vi "WLAN - TV - RW - ReadTestVectorFile(Tx).vi"(0 "TX_TV_Sequence":path[](array[path]), 5 "Measurment Settings":path[](array[path]), 13 "Index":i32) -> (4 "TV's":T2[](array[typedef]) {"Tx_Chan" format="%.0x"; "Standard" items=["80211A/G/J/P OFDM", "80211B/G DSSS", "80211G DSSSOFDM", "80211N MIMOOFDM", "80211AC MIMOOFDM"]; "OFDM Data Rate (Mbps)" items=["6", "9", "12", "18", "24", "36", "48", "54"]; "80211n PLCP Frame Format" items=["Mixed Format", "Greenfield Format"]; "FEC Coding Type" items=["BCC", "LDPC"]; "DSSS Data Rate (Mbps)" items=["1", "2", "5.5 CCK", "5.5 PBCC", "11 CCK", "11 PBCC", "22", "33"]}, 6 "Tv First Element":T2 {"Tx_Chan" format="%.0x"; "Standard" items=["80211A/G/J/P OFDM", "80211B/G DSSS", "80211G DSSSOFDM", "80211N MIMOOFDM", "80211AC MIMOOFDM"]; "OFDM Data Rate (Mbps)" items=["6", "9", "12", "18", "24", "36", "48", "54"]; "80211n PLCP Frame Format" items=["Mixed Format", "Greenfield Format"]; "FEC Coding Type" items=["BCC", "LDPC"]; "DSSS Data Rate (Mbps)" items=["1", "2", "5.5 CCK", "5.5 PBCC", "11 CCK", "11 PBCC", "22", "33"]}, 8 "Test Completed ?":bool, 10 "WLAN Measurement Settings":T3={"OFDM Advanced Controls(11ag)"={"OFDM Auto Compute Acquisition Length Enabled"=0, "OFDM Maximum Symbols Used"=0, "OFDM Time Tracking Enabled"=0, "OFDM Channel Tracking Enabled"=0, "OFDM Amplitude Tracking Enabled"=1, "OFDM CFO Estimation Method"=0, "OFDM Phase Tracking Method"=0, "OFDM Header Detection Enabled"=0, "OFDM MAC FCS Check Enabled"=0, "#Avg"=10, "#Iterations"=10}, "DSSS Demod Parameters"={"DSSS Auto Compute Acquisition Length Enabled"=0, "DSSS Equalization Enabled"=0, "DSSS Header Detection Enabled"=0, "DSSS MAC FCS Check Enabled"=0, "DSSS Measurement Start Location"=0, "DSSS Phase Tracking Method"=0, "DSSS Maximum Chips Used"=0, "DSSS Reference Pulse Shaping Filter"=0, "DSSS Reference Pulse Shaping Filter Coefficient"=0.0, "# Avg"=1024, "# Iterations"=1024, "DSSS Power Ramp Enabled"=0}, "OFDM Advanced Controls (11n)"={"OFDM Auto Compute Acquisition Length Enabled"=0, "OFDM Maximum Symbols Used"=0, "OFDM Time Tracking Enabled"=0, "OFDM Channel Tracking Enabled"=0, "OFDM Amplitude Tracking Enabled"=1, "OFDM CFO Estimation Method"=0, "OFDM Phase Tracking Method"=0, "OFDM Header Detection Enabled"=0, "OFDM MAC FCS Check Enabled"=0, "#Avg"=10, "#Iterations"=10}, "OFDM Advanced Controls(11ac)"={"OFDM Auto Compute Acquisition Length Enabled"=0, "OFDM Maximum Symbols Used"=0, "OFDM Time Tracking Enabled"=1, "OFDM Channel Tracking Enabled"=0, "OFDM Amplitude Tracking Enabled"=0, "OFDM CFO Estimation Method"=0, "OFDM Phase Tracking Method"=0, "OFDM Header Detection Enabled"=0, "OFDM MAC FCS Check Enabled"=0, "#Avg"=10, "#Iterations"=10}} {"OFDM Advanced Controls(11ac)"."OFDM Phase Tracking Method" items=["Standard", "Instantaneous", "None", "Standard with Cubic Spline Fit"]; "OFDM Advanced Controls(11ac)"."OFDM CFO Estimation Method" items=["Preamble Only", "Preamble and Data"]; "OFDM Advanced Controls(11ac)"."OFDM Channel Tracking Enabled" items=["False", "True"]; "OFDM Advanced Controls(11ac)"."OFDM Amplitude Tracking Enabled" items=["False", "True"]; "OFDM Advanced Controls(11ac)"."OFDM Time Tracking Enabled" items=["True"=1, "False"=0]; "OFDM Advanced Controls(11ac)"."OFDM Auto Compute Acquisition Length Enabled" items=["False", "True"]; "OFDM Advanced Controls(11ac)"."OFDM MAC FCS Check Enabled" items=["False", "True"]; "OFDM Advanced Controls(11ac)"."OFDM Header Detection Enabled" items=["False", "True"]; "OFDM Advanced Controls (11n)"."OFDM Phase Tracking Method" items=["Standard", "Instantaneous", "None", "Standard with Cubic Spline Fit"]; "OFDM Advanced Controls (11n)"."OFDM CFO Estimation Method" items=["Preamble Only", "Preamble and Data"]; "OFDM Advanced Controls (11n)"."OFDM Channel Tracking Enabled" items=["False", "True"]; "OFDM Advanced Controls (11n)"."OFDM Amplitude Tracking Enabled" items=["False", "True"]; "OFDM Advanced Controls (11n)"."OFDM Time Tracking Enabled" items=["True"=1, "False"=0]; "OFDM Advanced Controls (11n)"."OFDM Auto Compute Acquisition Length Enabled" items=["False", "True"]; "OFDM Advanced Controls (11n)"."OFDM MAC FCS Check Enabled" items=["False", "True"]; "OFDM Advanced Controls (11n)"."OFDM Header Detection Enabled" items=["False", "True"]; "DSSS Demod Parameters"."DSSS Power Ramp Enabled" items=["False", "True"]; "DSSS Demod Parameters"."DSSS Auto Compute Acquisition Length Enabled" items=["False", "True"]; "DSSS Demod Parameters"."DSSS Phase Tracking Method" items=["Standard", "Instantaneous"]; "DSSS Demod Parameters"."DSSS Equalization Enabled" items=["False", "True"]; "DSSS Demod Parameters"."DSSS Reference Pulse Shaping Filter" items=["Rectangular", "Raised Cosine", "Root Raised Cosine", "Gaussian"]; "DSSS Demod Parameters"."DSSS MAC FCS Check Enabled" items=["False", "True"]; "DSSS Demod Parameters"."DSSS Header Detection Enabled" items=["False", "True"]; "OFDM Advanced Controls(11ag)"."OFDM Phase Tracking Method" items=["Standard", "Instantaneous", "None", "Standard with Cubic Spline Fit"]; "OFDM Advanced Controls(11ag)"."OFDM CFO Estimation Method" items=["Preamble Only", "Preamble and Data"]; "OFDM Advanced Controls(11ag)"."OFDM Channel Tracking Enabled" items=["False", "True"]; "OFDM Advanced Controls(11ag)"."OFDM Amplitude Tracking Enabled" items=["False", "True"]; "OFDM Advanced Controls(11ag)"."OFDM Time Tracking Enabled" items=["True"=1, "False"=0]; "OFDM Advanced Controls(11ag)"."OFDM Auto Compute Acquisition Length Enabled" items=["False", "True"]; "OFDM Advanced Controls(11ag)"."OFDM MAC FCS Check Enabled" items=["False", "True"]; "OFDM Advanced Controls(11ag)"."OFDM Header Detection Enabled" items=["False", "True"]}, 14 "Cluster":T6)   [LabVIEW 2011]
uses:
  Includes/WLAN - TV - RW - INC - TV_DataType_Cluster.ctl
  Includes/WLAN - TV - RW - INC - Tx_Measurement_Cluster.ctl
  Includes/WLAN - TV - RW - INC - TV_OFDM Demod.ctl
  Includes/WLAN - TV - RW - INC - TV_DSSS Demod.ctl
  Includes/WLAN - TV - RW - INC - Tx_Measurement_Cluster(string).ctl
  Includes/WLAN - TV - RW - INC - Tx_Meas_Settings_OFDM_String.ctl
  Includes/WLAN - TV - RW - INC - Tx_Meas_Settings_DSSS_String.ctl
  Includes/WLAN - TV - RW - INC - TV_Parameters.ctl
  <vilib>/Utility/file.llb/Read From Spreadsheet File (string).vi
panel:
  in  "Tab Control":T1(tab)
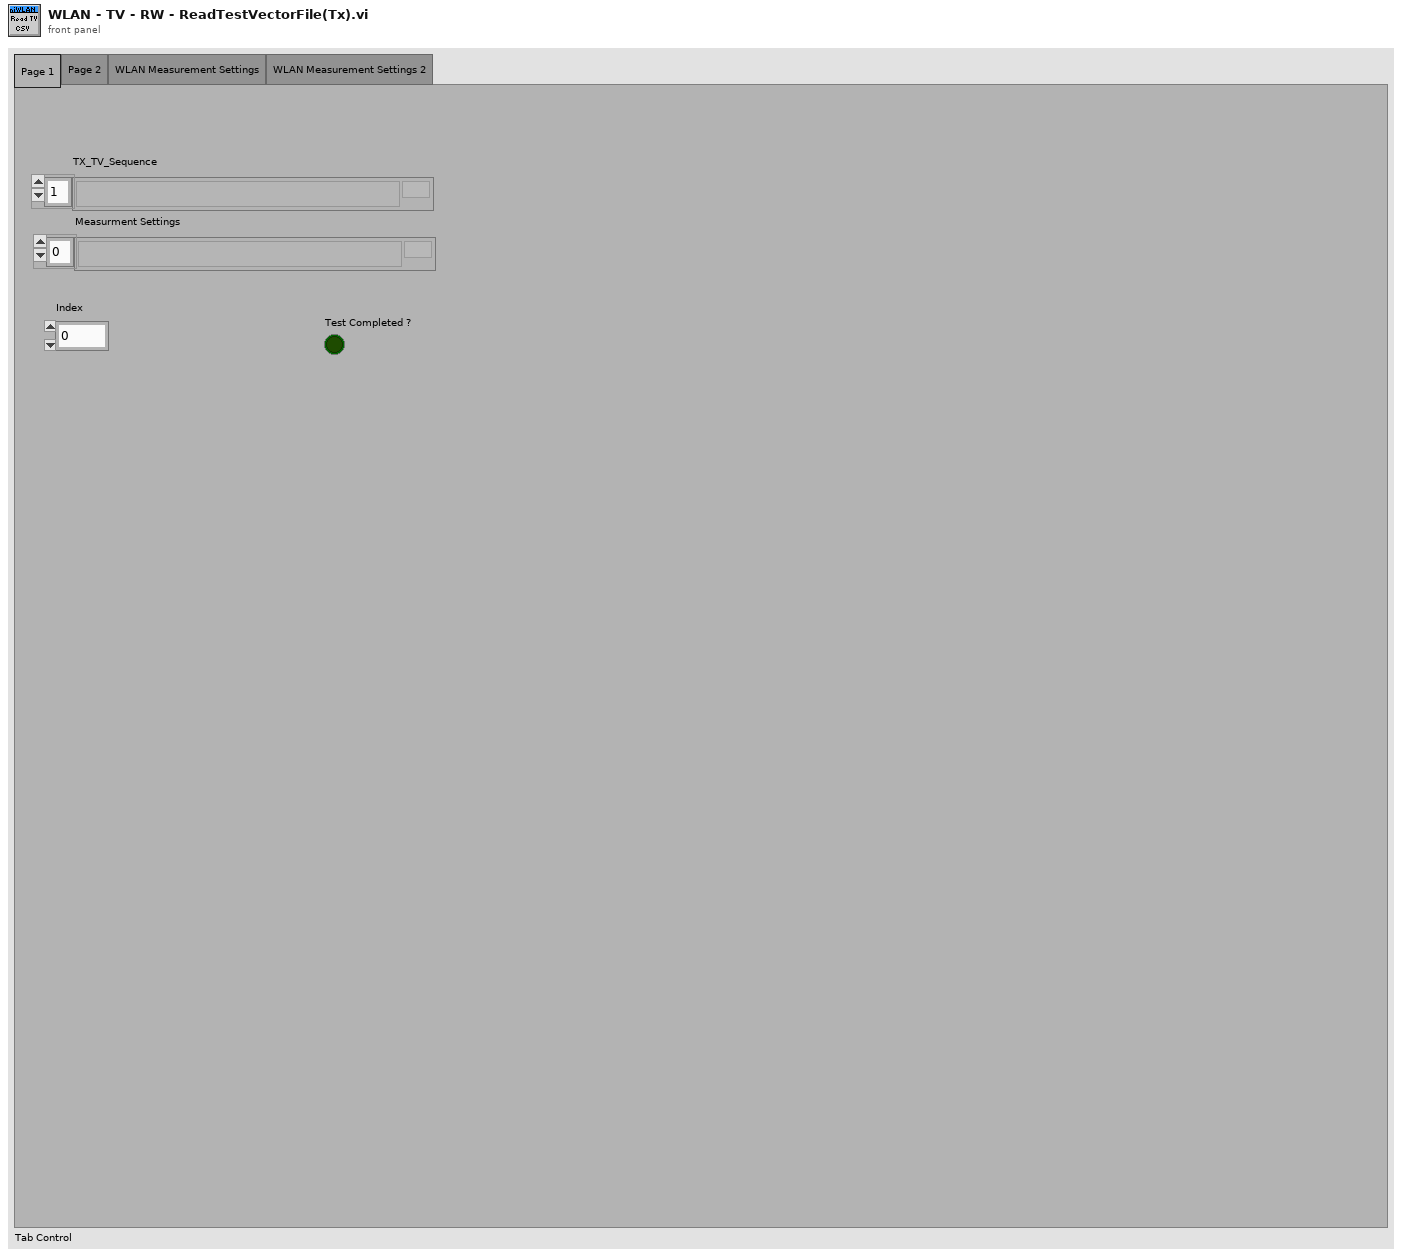
[diagram p1: front panel]
types:
  T1 = enum32{"Page 1", "Page 2", "WLAN Measurement Settings", "WLAN Measurement Settings 2"}
  T2 = typedef "WLAN - TV - RW - INC - TV_DataType_Cluster.ctl" = cluster{"Standard":i32, "Channel Frequency(Hz)":dbl, "Power Level(dBm)":dbl, "Channel Bandwidth (Hz)":dbl, "Idle Interval(s)":dbl, "OFDM Data Rate (Mbps)":i32, "OFDM Payload Length (bytes)":i32, "Number of Packets":i32, "MCS Index":i32, "Guard Interval (s)":dbl, "80211n PLCP Frame Format":i32, "FEC Coding Type":i32, "DSSS Data Rate (Mbps)":i32, "DSSS Payload Length (bytes)":i32, "N_SS":i32, "Tx_Chan":u32}
  T3 = typedef "WLAN - TV - RW - INC - Tx_Measurement_Cluster.ctl" = cluster{"OFDM Advanced Controls(11ag)":T4, "DSSS Demod Parameters":T5, "OFDM Advanced Controls (11n)":T4, "OFDM Advanced Controls(11ac)":cluster{"OFDM Auto Compute Acquisition Length Enabled":i32, "OFDM Maximum Symbols Used":i32, "OFDM Time Tracking Enabled":i32, "OFDM Channel Tracking Enabled":i32, "OFDM Amplitude Tracking Enabled":i32, "OFDM CFO Estimation Method":i32, "OFDM Phase Tracking Method":i32, "OFDM Header Detection Enabled":i32, "OFDM MAC FCS Check Enabled":i32, "#Avg":i32, "#Iterations":i32}}
  T4 = typedef "WLAN - TV - RW - INC - TV_OFDM Demod.ctl" = cluster{"OFDM Auto Compute Acquisition Length Enabled":i32, "OFDM Maximum Symbols Used":i32, "OFDM Time Tracking Enabled":i32, "OFDM Channel Tracking Enabled":i32, "OFDM Amplitude Tracking Enabled":i32, "OFDM CFO Estimation Method":i32, "OFDM Phase Tracking Method":i32, "OFDM Header Detection Enabled":i32, "OFDM MAC FCS Check Enabled":i32, "#Avg":i32, "#Iterations":i32}
  T5 = typedef "WLAN - TV - RW - INC - TV_DSSS Demod.ctl" = cluster{"DSSS Auto Compute Acquisition Length Enabled":i32, "DSSS Equalization Enabled":i32, "DSSS Header Detection Enabled":i32, "DSSS MAC FCS Check Enabled":i32, "DSSS Measurement Start Location":i32, "DSSS Phase Tracking Method":i32, "DSSS Maximum Chips Used":i32, "DSSS Reference Pulse Shaping Filter":i32, "DSSS Reference Pulse Shaping Filter Coefficient":dbl, "# Avg":i32, "# Iterations":i32, "DSSS Power Ramp Enabled":i32}
  T6 = typedef "WLAN - TV - RW - INC - Tx_Measurement_Cluster(string).ctl" = cluster{"OFDM Measurement Settings(11a)":T7, "TV Paramaters(11b)":T8, "OFDM Measurement Settings(11n) ":T7, "OFDM Measurement Settings(11ac) ":T7}
  T7 = typedef "WLAN - TV - RW - INC - Tx_Meas_Settings_OFDM_String.ctl" = cluster{"OFDM Auto Compute Acquisition Length Enabled":string, "OFDM Maximum Symbols Used":string, "OFDM Time Tracking Enabled":string, "OFDM Channel Tracking Enabled":string, "OFDM Amplitude Tracking Enabled":string, "OFDM CFO Estimation Method":string, "OFDM Phase Tracking Method":string, "OFDM Header Detection Enabled":string, "OFDM MAC FCS Check Enabled":string, "#Avg":string, "#Iterations":string}
  T8 = typedef "WLAN - TV - RW - INC - Tx_Meas_Settings_DSSS_String.ctl" = cluster{"DSSS Auto Compute Acquisition Length Enabled":string, "DSSS Equalization Enabled":string, "DSSS Header Detection Enabled":string, "DSSS MAC FCS Check Enabled":string, "DSSS Measurement Start Location":string, "DSSS Phase Tracking Method":string, "DSSS Maximum Chips Used":string, "DSSS Reference Pulse Shaping Filter":string, "DSSS Reference Pulse Shaping Filter Coefficient":string, "#Avg":string, "#Iterations":string, "DSSS Ramp Enabled ":string}
  T9 = typedef "WLAN - TV - RW - INC - TV_Parameters.ctl" = cluster{"Standard ":string, "Channel Frequency(Hz)":string, "Power Level(dBm)":string, "Channel Bandwidth (Hz)":string, "Idle Interval (s)":string, "OFDM Data Rate (Mbps)":string, "OFDM Payload Length (bytes)":string, "MCS Index":string, "Guard Interval (s)":string, "80211n PLCP Frame Format":string, "FEC Coding Type":string, "DSSS Data Rate (Mbps)":string, "DSSS Payload Length (bytes)":string, "#Packets":string, "N_SS":string, "Tx_Chan":string}
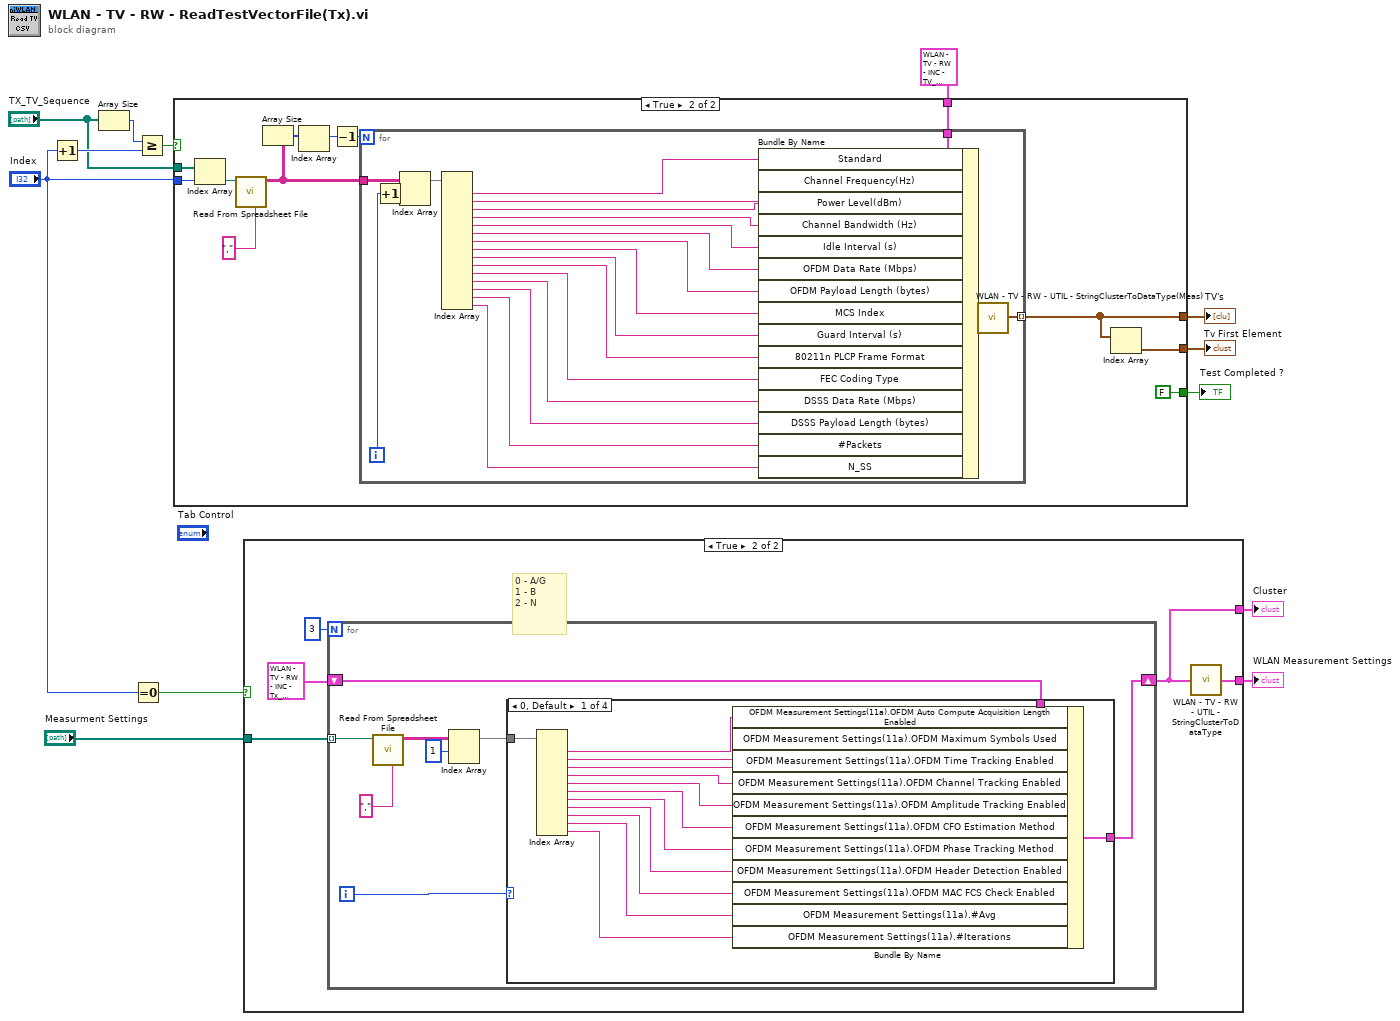
[diagram p0: block diagram]
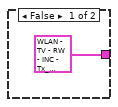
[diagram p2: hidden frame]
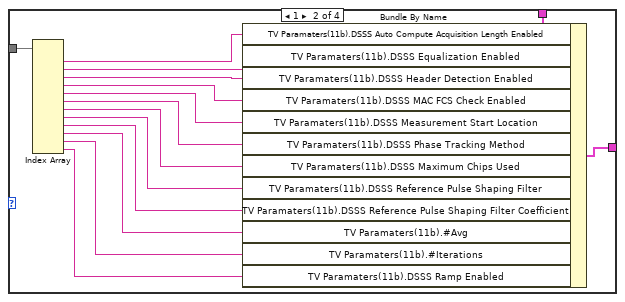
[diagram p3: hidden frame]
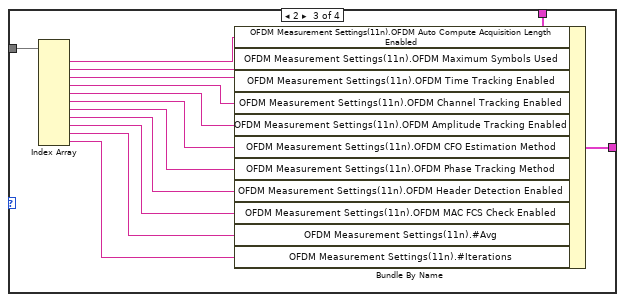
[diagram p4: hidden frame]
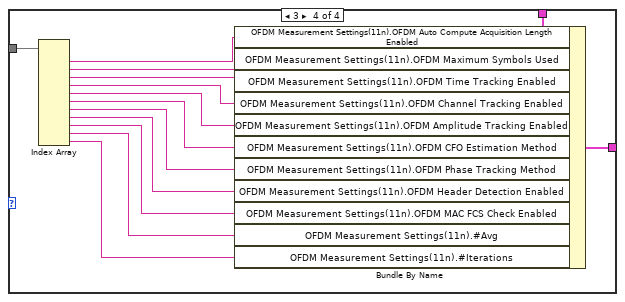
[diagram p5: hidden frame]
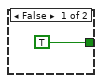
[diagram p6: hidden frame]
diagram:
  n1 = Increment(x="Index") -> (x+1=w10:i32)
  n2 = Array Size(array="TX_TV_Sequence") -> (size(s)=w11:i32)
  n3 = Equal To 0?(x="Index") -> (x = 0?=w4:bool)
  n4 = Greater Or Equal?(x=w11, y=w10) -> (x >= y?=w9:bool)
  n5 = case shown="True" w9 {
    tunnel: T9 {"Standard "="", "Channel Frequency(Hz)"="", "Power Level(dBm)"="", "Channel Bandwidth (Hz)"="", "Idle Interval (s)"="", "OFDM Data Rate (Mbps)"="", "OFDM Payload Length (bytes)"="", "MCS Index"="", "Guard Interval (s)"="", "80211n PLCP Frame Format"="", "FEC Coding Type"="", "DSSS Data Rate (Mbps)"="", "DSSS Payload Length (bytes)"="", "#Packets"="", "N_SS"="", "Tx_Chan"=""} ("TV Paramaters") -> [_ w25]
    tunnel: [_ w15] -> w12
    tunnel: "Index" -> [_ w23]
    tunnel: "TX_TV_Sequence" -> [_ w24]
    tunnel: [_ w21] -> w7
    tunnel: [TRUE ("Boolean") FALSE ("Boolean")] -> w6
    frame False {
    }
    frame True {
      n6 = Index Array(array=w24, index=w23) -> (element=w22:path)
      n7 = call-poly <vilib>:"Read From Spreadsheet File.vi"("delimiter (\\t)"="," ("delimiter (\\t)"), "file path (dialog if empty)"=w22) -> ("all rows"=w16:string[][])  [unwired: 5 in, 4 out]
      n8 = Array Size(array=w16) -> (size(s)=w19:i32[])
      n9 = Index Array(array=w19) -> (element=w18:i32)  [unwired: 1 in]
      n10 = Decrement(x=w18) -> (x-1=w17:i32)
      n11 = for {
        N: w17 -> [_]
        tunnel: w25 -> [w48]
        tunnel: [w32] -> w15 mode=indexing
        tunnel: w16 -> [w31]
        i -> [w29]
        n12 = Increment(x=w29) -> (x+1=w28:i32)
        n13 = Index Array(array=w31, index (row)=w28) -> (element=w30:string[])  [unwired: 1 in]
        n14 = Index Array(array=w30) -> (element #1=w47:string, element #2=w46:string, element #3=w45:string, element #4=w44:string, element #5=w43:string, element #6=w42:string, element #7=w41:string, element #8=w40:string, element #9=w39:string, element #10=w38:string, element #11=w37:string, element #12=w36:string, element #13=w35:string, element #14=w34:string, element #15=w27:string)  [unwired: 15 in]
        n15 = Bundle By Name(cluster=w48, "Standard"=w47, "Channel Frequency(Hz)"=w46, "Power Level(dBm)"=w45, "Channel Bandwidth (Hz)"=w44, "Idle Interval (s)"=w43, "OFDM Data Rate (Mbps)"=w42, "OFDM Payload Length (bytes)"=w41, "MCS Index"=w40, "Guard Interval (s)"=w39, "80211n PLCP Frame Format"=w38, "FEC Coding Type"=w37, "DSSS Data Rate (Mbps)"=w36, "DSSS Payload Length (bytes)"=w35, "#Packets"=w34, "N_SS"=w27) -> (w33:T9)
        n16 = call "WLAN - TV - RW - UTIL - StringClusterToDataType(Meas).vi"("TV Paramaters(String)"=w33) -> ("TV Parameters(DataType)"=w32:T2)  [unwired: 14 in]
      }
      n17 = Index Array(array=w15) -> (element=w21:T2)  [unwired: 1 in]
    }
  }
  "TV's" <- w12
  "Tv First Element" <- w7
  "Test Completed ?" <- w6
  n18 = case shown="True" w4 {
    tunnel: "Measurment Settings" -> [_ w54]
    tunnel: [T3 {"OFDM Advanced Controls(11ag)"={"OFDM Auto Compute Acquisition Length Enabled"=0, "OFDM Maximum Symbols Used"=0, "OFDM Time Tracking Enabled"=0, "OFDM Channel Tracking Enabled"=0, "OFDM Amplitude Tracking Enabled"=1, "OFDM CFO Estimation Method"=0, "OFDM Phase Tracking Method"=0, "OFDM Header Detection Enabled"=0, "OFDM MAC FCS Check Enabled"=0, "#Avg"=10, "#Iterations"=10}, "DSSS Demod Parameters"={"DSSS Auto Compute Acquisition Length Enabled"=0, "DSSS Equalization Enabled"=0, "DSSS Header Detection Enabled"=0, "DSSS MAC FCS Check Enabled"=0, "DSSS Measurement Start Location"=0, "DSSS Phase Tracking Method"=0, "DSSS Maximum Chips Used"=0, "DSSS Reference Pulse Shaping Filter"=0, "DSSS Reference Pulse Shaping Filter Coefficient"=0.0, "# Avg"=1024, "# Iterations"=1024, "DSSS Power Ramp Enabled"=0}, "OFDM Advanced Controls (11n)"={"OFDM Auto Compute Acquisition Length Enabled"=0, "OFDM Maximum Symbols Used"=0, "OFDM Time Tracking Enabled"=0, "OFDM Channel Tracking Enabled"=0, "OFDM Amplitude Tracking Enabled"=1, "OFDM CFO Estimation Method"=0, "OFDM Phase Tracking Method"=0, "OFDM Header Detection Enabled"=0, "OFDM MAC FCS Check Enabled"=0, "#Avg"=10, "#Iterations"=10}, "OFDM Advanced Controls(11ac)"={"OFDM Auto Compute Acquisition Length Enabled"=0, "OFDM Maximum Symbols Used"=0, "OFDM Time Tracking Enabled"=0, "OFDM Channel Tracking Enabled"=0, "OFDM Amplitude Tracking Enabled"=0, "OFDM CFO Estimation Method"=0, "OFDM Phase Tracking Method"=0, "OFDM Header Detection Enabled"=0, "OFDM MAC FCS Check Enabled"=0, "#Avg"=0, "#Iterations"=0}} ("WLAN Measurement Settings") w51] -> w2
    tunnel: [_ w50] -> w1
    frame False {
    }
    frame True {
      # "0 - A/G\n1 - B\n2 - N"
      n19 = for {
        N: 3 -> [_]
        tunnel: w54 -> [w62] mode=indexing
        shift-right: [w57] -> w50
        shift-left: T6 {"OFDM Measurement Settings(11a)"={"OFDM Auto Compute Acquisition Length Enabled"="", "OFDM Maximum Symbols Used"="", "OFDM Time Tracking Enabled"="", "OFDM Channel Tracking Enabled"="", "OFDM Amplitude Tracking Enabled"="", "OFDM CFO Estimation Method"="", "OFDM Phase Tracking Method"="", "OFDM Header Detection Enabled"="", "OFDM MAC FCS Check Enabled"="", "#Avg"="", "#Iterations"=""}, "TV Paramaters(11b)"={"DSSS Auto Compute Acquisition Length Enabled"="", "DSSS Equalization Enabled"="", "DSSS Header Detection Enabled"="", "DSSS MAC FCS Check Enabled"="", "DSSS Measurement Start Location"="", "DSSS Phase Tracking Method"="", "DSSS Maximum Chips Used"="", "DSSS Reference Pulse Shaping Filter"="", "DSSS Reference Pulse Shaping Filter Coefficient"="", "#Avg"="", "#Iterations"="", "DSSS Ramp Enabled "=""}, "OFDM Measurement Settings(11n) "={"OFDM Auto Compute Acquisition Length Enabled"="", "OFDM Maximum Symbols Used"="", "OFDM Time Tracking Enabled"="", "OFDM Channel Tracking Enabled"="", "OFDM Amplitude Tracking Enabled"="", "OFDM CFO Estimation Method"="", "OFDM Phase Tracking Method"="", "OFDM Header Detection Enabled"="", "OFDM MAC FCS Check Enabled"="", "#Avg"="", "#Iterations"=""}, "OFDM Measurement Settings(11ac) "={"OFDM Auto Compute Acquisition Length Enabled"="", "OFDM Maximum Symbols Used"="", "OFDM Time Tracking Enabled"="", "OFDM Channel Tracking Enabled"="", "OFDM Amplitude Tracking Enabled"="", "OFDM CFO Estimation Method"="", "OFDM Phase Tracking Method"="", "OFDM Header Detection Enabled"="", "OFDM MAC FCS Check Enabled"="", "#Avg"="", "#Iterations"=""}} ("Cluster") -> [w58]
        i -> [w56]
        n20 = call-poly <vilib>:"Read From Spreadsheet File.vi"("delimiter (\\t)"="," ("delimiter (\\t)"), "file path (dialog if empty)"=w62) -> ("all rows"=w60:string[][])  [unwired: 5 in, 4 out]
        n21 = Index Array(array=w60, index (row)=1) -> (element=w59:string[])  [unwired: 1 in]
        n22 = case shown="0, Default" w56 {
          tunnel: w59 -> [w76 w79 w105 w119]
          tunnel: w58 -> [w75 w78 w104 w118]
          tunnel: [w69 w77 w98 w112] -> w57
          frame 0, Default {
            n23 = Index Array(array=w76) -> (element #1=w74:string, element #2=w73:string, element #3=w72:string, element #4=w71:string, element #5=w70:string, element #6=w68:string, element #7=w67:string, element #8=w66:string, element #9=w65:string, element #10=w64:string, element #11=w63:string)  [unwired: 11 in]
            n24 = Bundle By Name(cluster=w75, "OFDM Measurement Settings(11a).OFDM Auto Compute Acquisition Length Enabled"=w74, "OFDM Measurement Settings(11a).OFDM Maximum Symbols Used"=w73, "OFDM Measurement Settings(11a).OFDM Time Tracking Enabled"=w72, "OFDM Measurement Settings(11a).OFDM Channel Tracking Enabled"=w71, "OFDM Measurement Settings(11a).OFDM Amplitude Tracking Enabled"=w70, "OFDM Measurement Settings(11a).OFDM CFO Estimation Method"=w68, "OFDM Measurement Settings(11a).OFDM Phase Tracking Method"=w67, "OFDM Measurement Settings(11a).OFDM Header Detection Enabled"=w66, "OFDM Measurement Settings(11a).OFDM MAC FCS Check Enabled"=w65, "OFDM Measurement Settings(11a).#Avg"=w64, "OFDM Measurement Settings(11a).#Iterations"=w63) -> (w69:T6)
          }
          frame 1 {
            n25 = Index Array(array=w79) -> (element #1=w91:string, element #2=w90:string, element #3=w89:string, element #4=w88:string, element #5=w87:string, element #6=w86:string, element #7=w85:string, element #8=w84:string, element #9=w83:string, element #10=w82:string, element #11=w81:string, element #12=w80:string)  [unwired: 12 in]
            n26 = Bundle By Name(cluster=w78, "TV Paramaters(11b).DSSS Auto Compute Acquisition Length Enabled"=w91, "TV Paramaters(11b).DSSS Equalization Enabled"=w90, "TV Paramaters(11b).DSSS Header Detection Enabled"=w89, "TV Paramaters(11b).DSSS MAC FCS Check Enabled"=w88, "TV Paramaters(11b).DSSS Measurement Start Location"=w87, "TV Paramaters(11b).DSSS Phase Tracking Method"=w86, "TV Paramaters(11b).DSSS Maximum Chips Used"=w85, "TV Paramaters(11b).DSSS Reference Pulse Shaping Filter"=w84, "TV Paramaters(11b).DSSS Reference Pulse Shaping Filter Coefficient"=w83, "TV Paramaters(11b).#Avg"=w82, "TV Paramaters(11b).#Iterations"=w81, "TV Paramaters(11b).DSSS Ramp Enabled"=w80) -> (w77:T6)
          }
          frame 2 {
            n27 = Index Array(array=w105) -> (element #1=w103:string, element #2=w102:string, element #3=w101:string, element #4=w100:string, element #5=w99:string, element #6=w97:string, element #7=w96:string, element #8=w95:string, element #9=w94:string, element #10=w93:string, element #11=w92:string)  [unwired: 11 in]
            n28 = Bundle By Name(cluster=w104, "OFDM Measurement Settings(11n).OFDM Auto Compute Acquisition Length Enabled"=w103, "OFDM Measurement Settings(11n).OFDM Maximum Symbols Used"=w102, "OFDM Measurement Settings(11n).OFDM Time Tracking Enabled"=w101, "OFDM Measurement Settings(11n).OFDM Channel Tracking Enabled"=w100, "OFDM Measurement Settings(11n).OFDM Amplitude Tracking Enabled"=w99, "OFDM Measurement Settings(11n).OFDM CFO Estimation Method"=w97, "OFDM Measurement Settings(11n).OFDM Phase Tracking Method"=w96, "OFDM Measurement Settings(11n).OFDM Header Detection Enabled"=w95, "OFDM Measurement Settings(11n).OFDM MAC FCS Check Enabled"=w94, "OFDM Measurement Settings(11n).#Avg"=w93, "OFDM Measurement Settings(11n).#Iterations"=w92) -> (w98:T6)
          }
          frame 3 {
            n29 = Index Array(array=w119) -> (element #1=w117:string, element #2=w116:string, element #3=w115:string, element #4=w114:string, element #5=w113:string, element #6=w111:string, element #7=w110:string, element #8=w109:string, element #9=w108:string, element #10=w107:string, element #11=w106:string)  [unwired: 11 in]
            n30 = Bundle By Name(cluster=w118, "OFDM Measurement Settings(11n).OFDM Auto Compute Acquisition Length Enabled"=w117, "OFDM Measurement Settings(11n).OFDM Maximum Symbols Used"=w116, "OFDM Measurement Settings(11n).OFDM Time Tracking Enabled"=w115, "OFDM Measurement Settings(11n).OFDM Channel Tracking Enabled"=w114, "OFDM Measurement Settings(11n).OFDM Amplitude Tracking Enabled"=w113, "OFDM Measurement Settings(11n).OFDM CFO Estimation Method"=w111, "OFDM Measurement Settings(11n).OFDM Phase Tracking Method"=w110, "OFDM Measurement Settings(11n).OFDM Header Detection Enabled"=w109, "OFDM Measurement Settings(11n).OFDM MAC FCS Check Enabled"=w108, "OFDM Measurement Settings(11n).#Avg"=w107, "OFDM Measurement Settings(11n).#Iterations"=w106) -> (w112:T6)
          }
        }
      }
      n31 = call "WLAN - TV - RW - UTIL - StringClusterToDataType.vi"("TV Paramaters(String)"=w50) -> ("WLAN Measurement Settings"=w51:T3)  [unwired: 14 in]
    }
  }
  "WLAN Measurement Settings" <- w2
  "Cluster" <- w1
